vi "Strip Path.vi"(11 "Path String":string) -> (2 "Stripped Segment":string, 3 "Remaining Path":string)   [LabVIEW 2020, in "URI.lvlib"]
uses:
  URI.lvlib
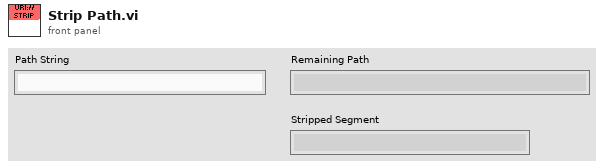
[diagram p1: front panel]
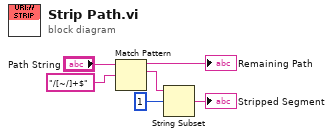
[diagram p0: block diagram]
diagram:
  n1 = Match Pattern(string="Path String", regular expression="/[~/]+$") -> (before substring=→"Remaining Path":string, match substring=w4:string)  [unwired: 1 in, 2 out]
  n2 = String Subset(string=w4, offset (0)=1) -> (substring=→"Stripped Segment":string)  [unwired: 1 in]
